vi "GetEventHardpointMonitorStateField.vi"(10 "Event Data":string, 11 "Cluster in":refnum<vi>) -> (3 "Array":string[](array[string]))   [LabVIEW 2016]
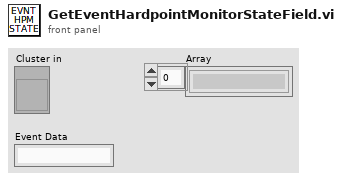
[diagram p1: front panel]
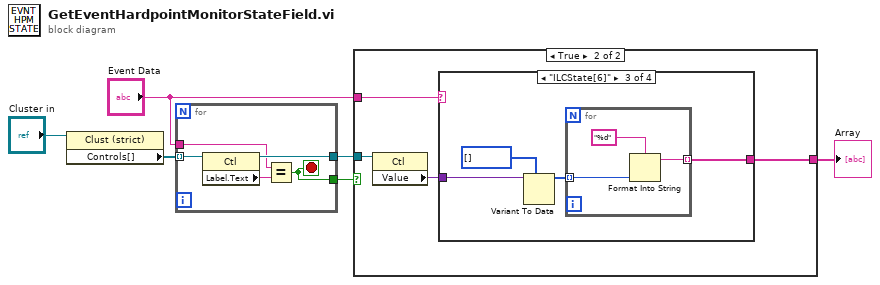
[diagram p0: block diagram]
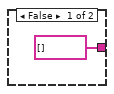
[diagram p2: hidden frame]
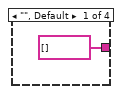
[diagram p3: hidden frame]
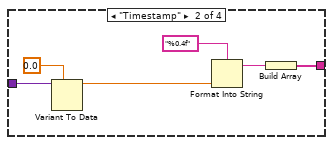
[diagram p4: hidden frame]
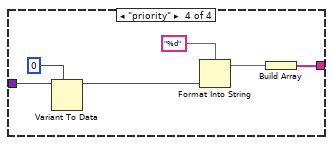
[diagram p5: hidden frame]
diagram:
  n1 = property on="Property Node" class="Clust (strict)"(reference="Cluster in") -> ("Controls[]"=w3:refnum<vi>[])  [unwired: 1 in, 2 out]
  n2 = for {
    tunnel: w3 -> [w11] mode=indexing
    tunnel: [w10] -> w5
    tunnel: "Event Data" -> [w8]
    tunnel: [w7] -> w6
    stop <- w7 stop-if-true
    n3 = property on="Property Node" class="Ctl"(reference=w11) -> (reference out=w10:refnum<vi>, "Label.Text"=w9:string)  [unwired: 1 in, 1 out]
    n4 = Equal?(x=w8, y=w9) -> (x = y?=w7:bool)
  }
  n5 = case shown="True" w6 {
    tunnel: "Event Data" -> [_ w16]
    tunnel: w5 -> [_ w15]
    tunnel: [string[] [] w13] -> w2
    frame False {
    }
    frame True {
      n6 = property on="Property Node" class="Ctl"(reference=w15) -> ("Value"=w14:variant)  [unwired: 1 in, 2 out]
      n7 = case shown="\"ILCState[6]\"" w16 {
        tunnel: [string[] [] w21 w24 w34] -> w13
        tunnel: w14 -> [_ w19 w27 w32]
        frame "", Default {
        }
        frame "Timestamp" {
          n8 = Variant To Data(type=0.0, Variant=w19) -> (data=w20:dbl)  [unwired: 1 in, 1 out]
          n9 = Format Into String(format string="%0.4f", w20) -> (resulting string=w22:string)  [unwired: 2 in, 1 out]
          n10 = Build Array(w22) -> (w21:string[])
        }
        frame "ILCState[6]" {
          n11 = Variant To Data(type=i16[] [], Variant=w27) -> (data=w25:i16[])  [unwired: 1 in, 1 out]
          n12 = for {
            tunnel: w25 -> [w29] mode=indexing
            tunnel: [w28] -> w24 mode=indexing
            n13 = Format Into String(format string="%d", w29) -> (resulting string=w28:string)  [unwired: 2 in, 1 out]
          }
        }
        frame "priority" {
          n14 = Variant To Data(type=0, Variant=w32) -> (data=w33:i32)  [unwired: 1 in, 1 out]
          n15 = Format Into String(format string="%d", w33) -> (resulting string=w35:string)  [unwired: 2 in, 1 out]
          n16 = Build Array(w35) -> (w34:string[])
        }
      }
    }
  }
  "Array" <- w2
